vi "StopSweeps.vi"(8 "error in (no error)":errorcluster, 11 "config":T1) -> (0 "error out":errorcluster, 3 "config out":T1)   [LabVIEW 2017, in "EmsaAcquisition.lvlib"]
uses:
  <vilib>/addons/InsightCM/Devices/Shared/Emsa/EmsaAcquisition/EmsaAcquisition.lvlib
  <vilib>/addons/InsightCM/Devices/Shared/Emsa/EmsaAcquisition/controls/config.ctl
  <vilib>/addons/InsightCM/Devices/Shared/Emsa/Emsa9770API/9770 API.lvclass
  <vilib>/addons/InsightCM/Devices/Shared/Emsa/EmsaAcquisition/controls/group.ctl
  <vilib>/addons/InsightCM/Devices/Shared/Emsa/EmsaAcquisition/controls/acqConfig.ctl
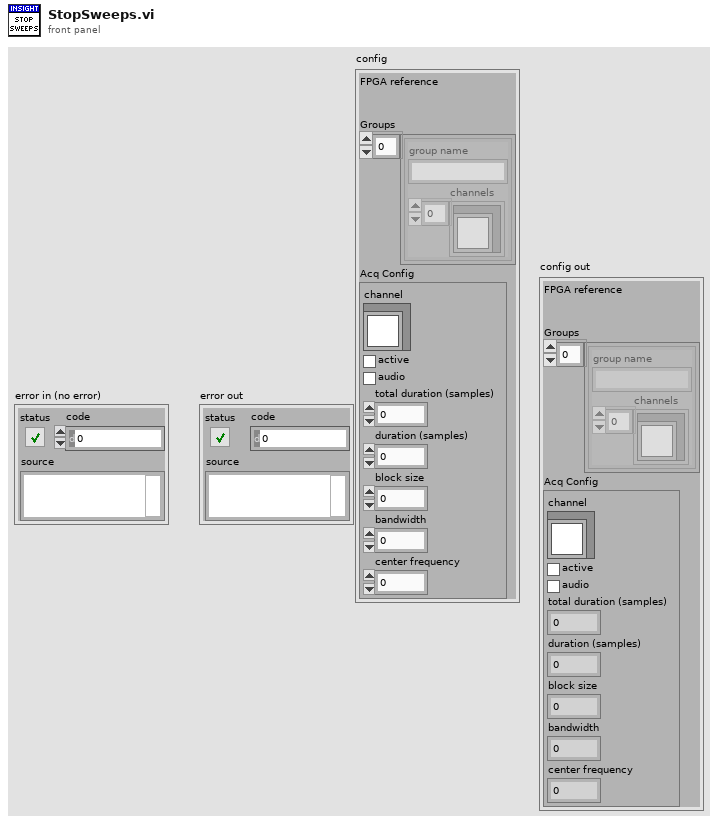
[diagram p1: front panel]
types:
  T1 = typedef "EmsaAcquisition.lvlib/config.ctl" = cluster{"FPGA reference":refnum<k20>, "Groups":T2[], "Acq Config":T3}
  T2 = typedef "EmsaAcquisition.lvlib/group.ctl" = cluster{"group name":string, "channels":refnum<class "9770 API.lvclass">[]}
  T3 = typedef "EmsaAcquisition.lvlib/acqConfig.ctl" = cluster{"channel":refnum<class "9770 API.lvclass">, "active":bool, "audio":bool, "total duration (samples)":i32, "duration (samples)":i32, "block size":i32, "bandwidth":dbl, "center frequency":dbl}
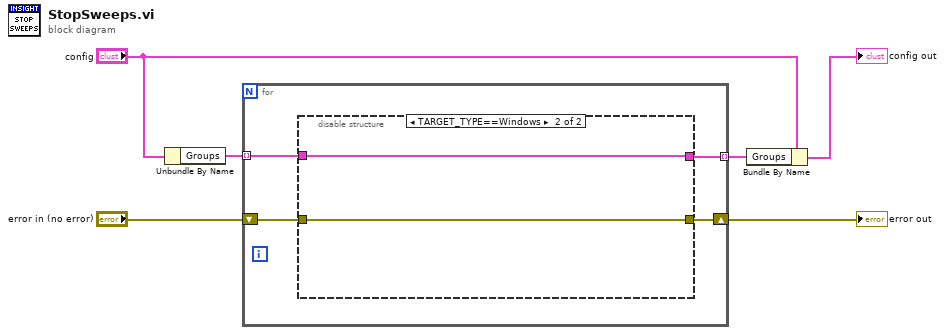
[diagram p0: block diagram]
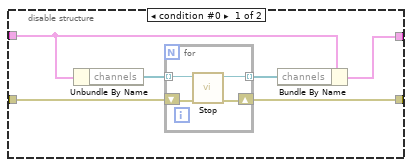
[diagram p2: hidden frame]
diagram:
  n1 = Unbundle By Name("config") -> ("Groups"=w4:T2[])
  n2 = for {
    tunnel: w4 -> [w8] mode=indexing
    shift-right: [w9] -> w5
    shift-left: "error in (no error)" -> [w10]
    tunnel: [w7] -> w3 mode=indexing
    n3 = disable-structure shown="TARGET_TYPE==Windows" {
      disable-tunnel: w10 -> [w16 w21]
      disable-tunnel: [w14 w21] -> w9
      disable-tunnel: w8 -> [w13 w22]
      disable-tunnel: [w11 w22] -> w7
      frame condition #0 {
        n4 = Unbundle By Name(w13) -> ("channels"=w15:refnum<class "9770 API.lvclass">[])
        n5 = for {
          shift-right: [w19] -> w14
          shift-left: w16 -> [w18]
          tunnel: w15 -> [w20] mode=indexing
          tunnel: [w17] -> w12 mode=indexing
          n6 = call-dynamic "Stop.vi"("error in (no error)"=w18, "RIO_API in"=w20) -> ("error out"=w19:errorcluster, "RIO_API out"=w17:refnum<class "9770 API.lvclass">)  [unwired: 8 in]
        }
        n7 = Bundle By Name(cluster=w13, "channels"=w12) -> (w11:T2)
      }
      frame condition #1 (active) {
      }
    }
  }
  "error out" <- w5
  n8 = Bundle By Name(cluster="config", "Groups"=w3) -> (→"config out":T1)
